vi "test Properties.vi"(8 "error in (no error)":errorcluster, 11 "TestCase in":refnum<class "Test_Queue.lvclass">) -> (0 "error out":errorcluster, 3 "TestCase out":refnum<class "Test_Queue.lvclass">)   [LabVIEW 2015, in "Test_Queue.lvclass"]
uses:
  Test_Queue.lvclass
  Global Parameters.vi
  Core/Session/Session.lvclass
  Queue/NI_Azure_Queue.lvlib
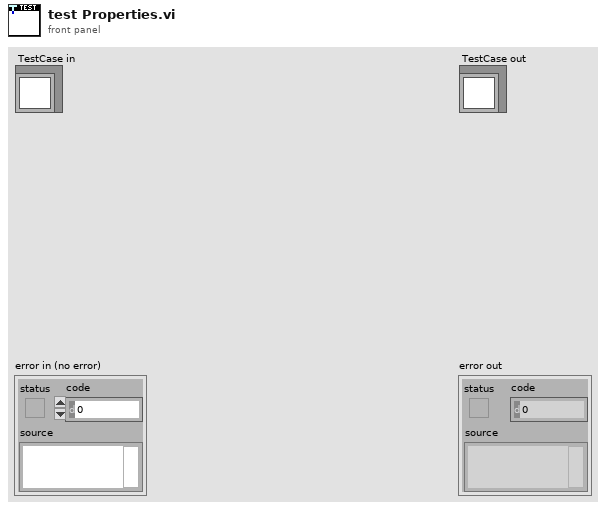
[diagram p1: front panel]
types:
  T1 = typedef "NI_Azure_Core.lvlib/Session.lvclass/Azure Credentials.ctl" = cluster{"Storage Account Name":string, "Access Key":string}
  T2 = typedef "NI_Azure_Queue.lvlib/Queue Service Properties.ctl" = cluster{"Logging":T3, "Hour metrics":T5, "Minute metrics":T5, "Cors rule":T6}
  T3 = typedef "NI_Azure_Queue.lvlib/Logging.ctl" = cluster{"Version":dbl, "Delete":bool, "Read":bool, "Write":bool, "Retention policy":T4}
  T4 = typedef "NI_Azure_Queue.lvlib/Retention Policy.ctl" = cluster{"Enabled":bool, "Days":u32}
  T5 = typedef "NI_Azure_Queue.lvlib/Metrics.ctl" = cluster{"Version":dbl, "Enabled":bool, "Include APIs":bool, "Retention policy":T4}
  T6 = typedef "NI_Azure_Queue.lvlib/Cors Rule.ctl" = cluster{"Allowed origins":string[], "Allowed methods":string[], "Max Age (s)":u32, "Exposed headers":string[], "Allowed headers":string[]}
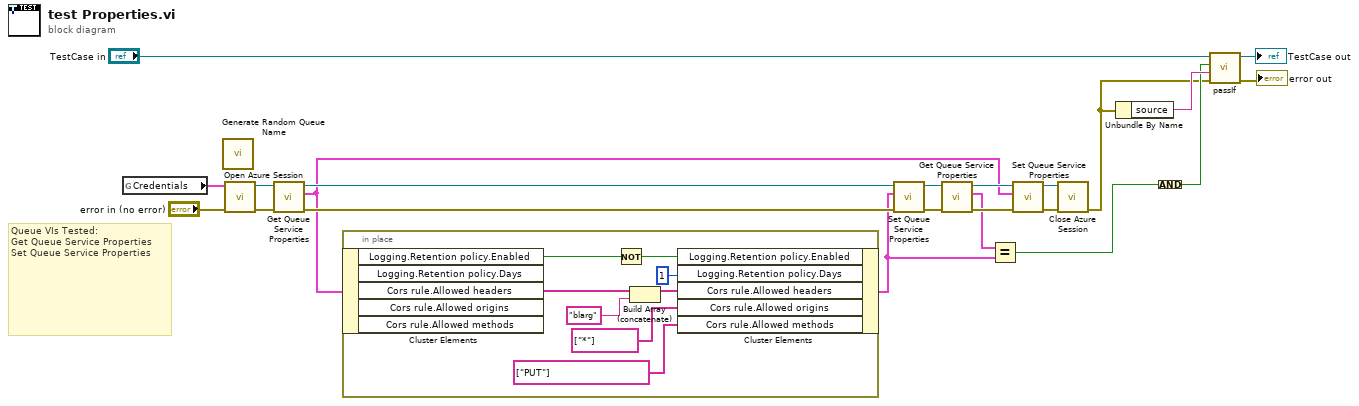
[diagram p0: block diagram]
diagram:
  # "Queue VIs Tested:\nGet Queue Service Properties\nSet Queue Service Properties"
  n1 = global read "Global Parameters.vi" "Credentials"() -> (w16:T1)
  n2 = call "Generate Random Queue Name.vi"() -> ()  [unwired: 11 in, 1 out]
  n3 = call "Open Azure Session.vi"("error in (no error)"="error in (no error)", "Credentials"=w16) -> ("error out"=w17:errorcluster, "Azure Session"=w14:refnum<class "Session.lvclass">)  [unwired: 8 in]
  n4 = call "Get Queue Service Properties.vi"("error in (no error)"=w17, "Azure Session in"=w14) -> ("error out"=w12:errorcluster, "Queue Service Properties"=w2:T2, "Azure Session out"=w10:refnum<class "Session.lvclass">)  [unwired: 7 in]
  n5 = in-place {
    n6 = in-place-cluster #1(w2) -> ("Logging.Retention policy.Enabled"=w30:bool, "Cors rule.Allowed headers"=w27:string[])  [unwired: 3 out]
    n7 = Not(x=w30) -> (.not. x?=w29:bool)
    n8 = Build Array (concatenate)(w27, "blarg") -> (w26:string[])
    n9 = in-place-cluster #1("Logging.Retention policy.Enabled"=w29, "Logging.Retention policy.Days"=u32 1, "Cors rule.Allowed headers"=w26, "Cors rule.Allowed origins"=string[] ["*"], "Cors rule.Allowed methods"=string[] ["PUT"]) -> (w6:T2)
  }
  n10 = call "Set Queue Service Properties.vi"("error in (no error)"=w12, "Queue Service Properties"=w6, "Azure Session in"=w10) -> ("error out"=w11:errorcluster, "Azure Session out"=w8:refnum<class "Session.lvclass">)  [unwired: 7 in]
  n11 = call "Get Queue Service Properties.vi"("error in (no error)"=w11, "Azure Session in"=w8) -> ("error out"=w9:errorcluster, "Queue Service Properties"=w7:T2, "Azure Session out"=w3:refnum<class "Session.lvclass">)  [unwired: 7 in]
  n12 = Equal?(x=w7, y=w6) -> (x = y?=w5:bool)
  n13 = call "Set Queue Service Properties.vi"("error in (no error)"=w9, "Queue Service Properties"=w2, "Azure Session in"=w3) -> ("error out"=w4:errorcluster, "Azure Session out"=w1:refnum<class "Session.lvclass">)  [unwired: 7 in]
  n14 = call "Close Azure Session.vi"("error in (no error)"=w4, "Azure Session"=w1) -> ("error out"=w13:errorcluster)  [unwired: 9 in]
  n15 = Unbundle By Name(w13) -> ("source"=w19:string)
  n16 = Compound Arithmetic op=AND(w5) -> (w15:bool)
  n17 = call-dynamic "passIf.vi"("error in (no error)"=w13, "message (\"\")"=w19, "pass"=w15, "TestCase in"="TestCase in") -> ("error out"=→"error out":errorcluster, "TestCase out"=→"TestCase out":refnum<class "Test_Queue.lvclass">)  [unwired: 6 in]
